vi "Insert Test.vi"(4 "Unique ID":string, 6 "Insertion Index":i32=-1, 7 "Parent ID":string, 8 "error in (no error)":errorcluster, 9 "Test":refnum<class "Executioner.lvclass">, 10 "Name":string, 11 "Test Executive in":refnum<class "Test Executive.lvclass">) -> (0 "error out":errorcluster, 1 "Replaced?":bool, 2 "Unique ID out":string, 3 "Test Executive out":refnum<class "Test Executive.lvclass">)   [LabVIEW 2019, in "Test Executive.lvlib" / "Test Executive.lvclass"]
uses:
  <vilib>/gpm_packages/@cs/test-executive/Source/Test Executive/TestExecutive/Test Executive.lvclass
  <vilib>/gpm_packages/@cs/test-executive/Source/Test Executive/Executioner/Executioner.lvclass
  <vilib>/gpm_packages/@cs/test-executive/Source/Test Executive/TestExecutive/Test Executive.lvclass/Test Executive.ctl
  <vilib>/gpm_packages/@cs/linked-list/Source/Linked List/Linked List Ref/Linked List Ref.lvclass
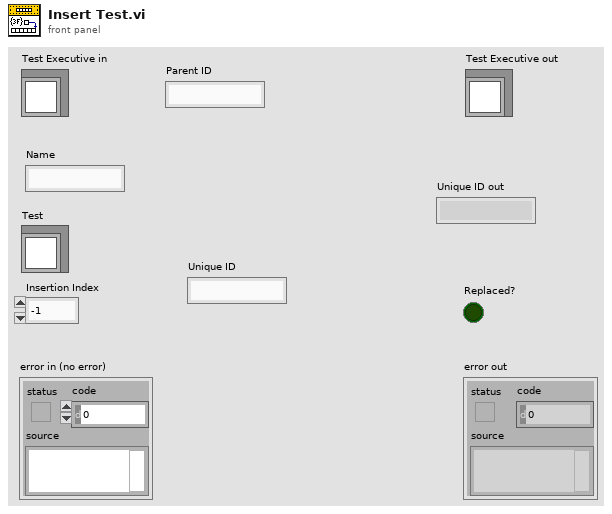
[diagram p1: front panel]
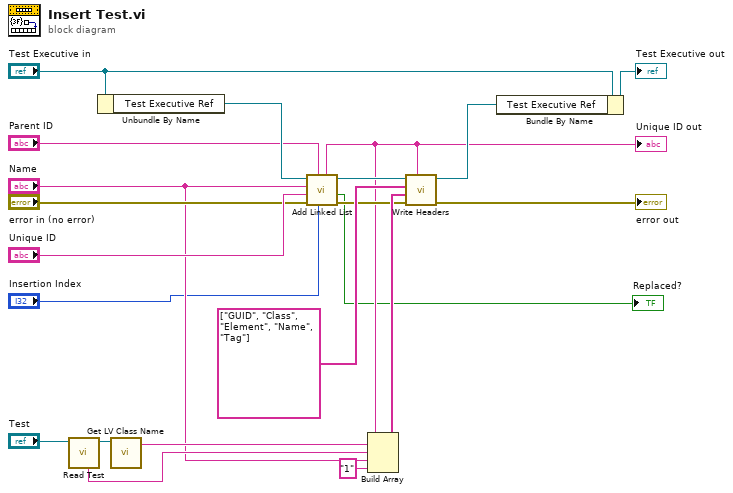
[diagram p0: block diagram]
diagram:
  n1 = call <vilib>:"Read Test.vi"("Executioner in"="Test") -> ("Executioner out"=w14:refnum<class "Executioner.lvclass">, "Test"=w12:string)  [unwired: 9 in]
  n2 = Unbundle By Name("Test Executive in") -> ("Test Executive Ref"=w21:refnum<data-value>)
  n3 = call <vilib>:"Get LV Class Name.vi"("object"=w14) -> ("class name"=w13:string)  [unwired: 9 in, 1 out]
  n4 = call <vilib>:"Add Linked List.vi"("Insertion Index"="Insertion Index", "Parent ID"="Parent ID", "error in (no error)"="error in (no error)", "Linked List ID"="Unique ID", "Name"="Name", "Linked List Ref"=w21) -> ("error out"=w8:errorcluster, "Replaced?"=→"Replaced?":bool, "Linked List Ref out"=w17:refnum<data-value>, "Linked List ID out"=w3:string)  [unwired: 2 in]
  "Unique ID out" <- w3
  n5 = Build Array(w3, w13, w12, "Name", "1" ("element")) -> (w9:string[])
  n6 = call <vilib>:"Write Headers.vi"("Linked List ID"=w3, "error in (no error)"=w8, "Header Values"=w9, "Header Names"=string[] ["GUID", "Class", "Element", "Name", "Tag"], "Linked List Ref"=w17) -> ("error out"=→"error out":errorcluster, "Linked List Ref out"=w6:refnum<data-value>)  [unwired: 5 in]
  n7 = Bundle By Name(cluster="Test Executive in", "Test Executive Ref"=w6) -> (→"Test Executive out":refnum<class "Test Executive.lvclass">)
